vi "SQL_Query.vi"(0 "SQL in":refnum<class "SQL.lvclass">, 1 "Column to compare":i32=1, 5 "Compare":string, 9 "Table":string, 11 "error in (no error)":errorcluster) -> (4 "SQL out":refnum<class "SQL.lvclass">, 6 "Found?":bool, 8 "Compare":string, 15 "error out":errorcluster)   [LabVIEW 2012, in "SQL.lvclass"]
uses:
  SQL.lvclass
  <vilib>/addons/database/_DB Variant To Data/Database Variant To Data.xnode
  <vilib>/addons/database/NI_Database_API.lvlib
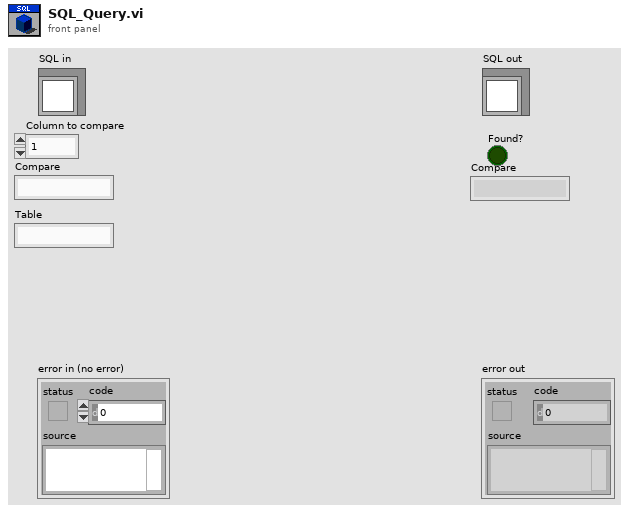
[diagram p1: front panel]
types:
  T1 = typedef "SQL.lvclass/ObjectAttributes.ctl" = cluster{"DB Connection Reference":T2}
  T2 = typedef "NI_Database_API.lvlib/Conn ObjectReference.ctl" = refnum<k1>
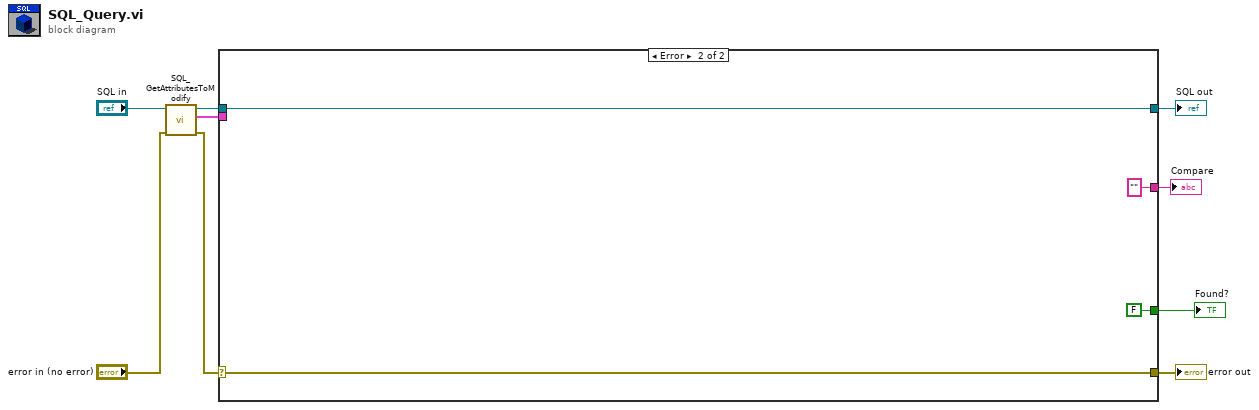
[diagram p0: block diagram]
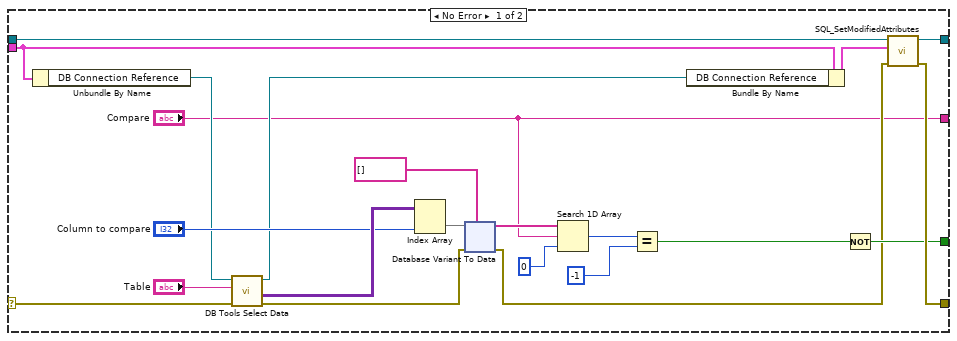
[diagram p2: hidden frame]
diagram:
  n1 = call "SQL_GetAttributesToModify.vi"("error in (no error)"="error in (no error)", "reference in"="SQL in") -> ("error out"=w4:errorcluster, "Attributes"=w3:T1, "reference out"=w6:refnum<class "SQL.lvclass">)  [unwired: 6 in, 1 out]
  n2 = case shown="Error" w4 {
    selector: w4 -> [w28 w73]
    tunnel: [w29 w73] -> w9
    tunnel: [w30 w72] -> w8
    tunnel: w6 -> [w31 w72]
    tunnel: w3 -> [w17 _]
    tunnel: [w18 FALSE] -> w2
    tunnel: ["Compare" "" ("Compare")] -> w1
    frame No Error {
      n3 = Unbundle By Name(w17) -> ("DB Connection Reference"=w15:T2)
      n4 = call <vilib>:"DB Tools Select Data.vi"("error in (no error)"=w28, "table"="Table", "connection reference"=w15) -> ("error out"=w24:errorcluster, "data"=w27:variant[][], "connection reference out"=w14:T2)  [unwired: 3 in]
      n5 = Index Array(array=w27, index (col)="Column to compare") -> (element=w12:variant[])  [unwired: 1 in]
      n6 = xnode "Database Variant To Data"("database variant"=w12, "error in (no error)"=w24, "type"=string[] []) -> ("data"=w13:string[], "error out"=w11:errorcluster)
      n7 = Search 1D Array(1D array=w13, element="Compare", start index (0)=0) -> (index of element=w23:i32)
      n8 = Equal?(x=w23, y=-1) -> (x = y?=w19:bool)
      n9 = Bundle By Name(cluster=w17, "DB Connection Reference"=w14) -> (w16:T1)
      n10 = Not(x=w19) -> (.not. x?=w18:bool)
      n11 = call "SQL_SetModifiedAttributes.vi"("error in (no error)"=w11, "Attributes"=w16, "reference in"=w31) -> ("error out"=w29:errorcluster, "reference out"=w30:refnum<class "SQL.lvclass">)  [unwired: 7 in]
    }
    frame Error {
    }
  }
  "error out" <- w9
  "SQL out" <- w8
  "Found?" <- w2
  "Compare" <- w1
